vi "读D字符转数值.vi"(10 "读取D个数":i32=1 min=0 max=10, 11 "读取D地址":i32) -> (2 "读取的字节数":i32, 3 "连接的字符串":string)   [LabVIEW 2012]
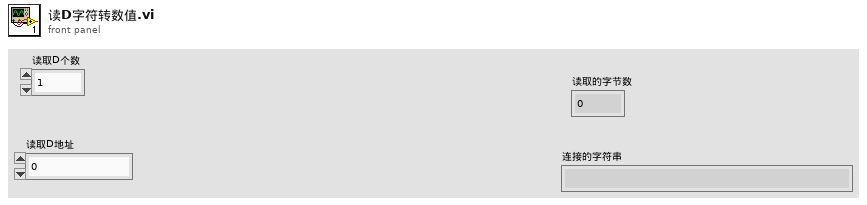
[diagram p1: front panel]
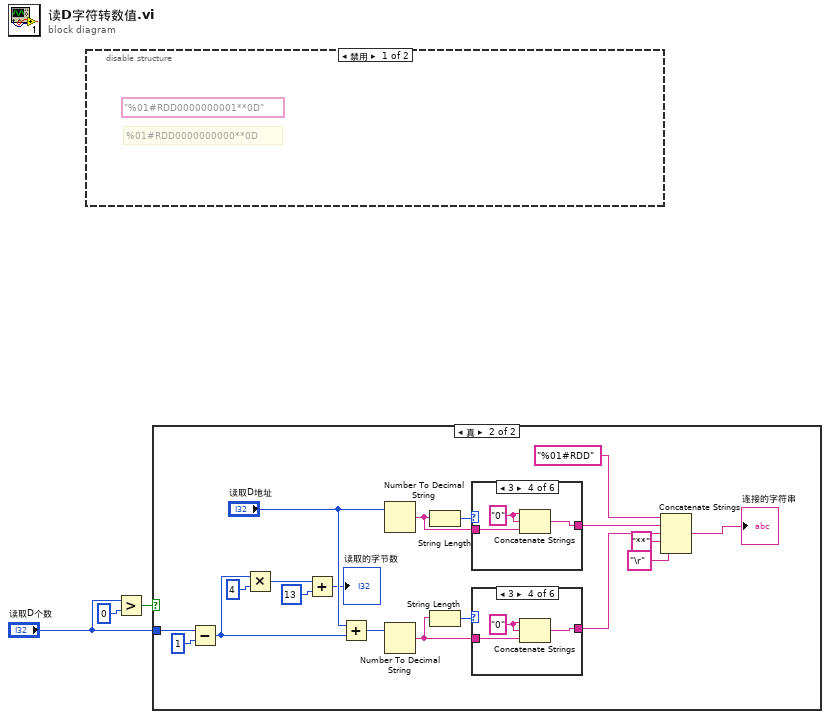
[diagram p0: block diagram]
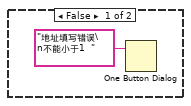
[diagram p2: hidden frame]
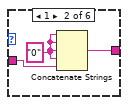
[diagram p4: hidden frame]
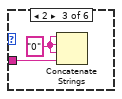
[diagram p5: hidden frame]
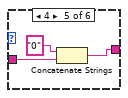
[diagram p6: hidden frame]
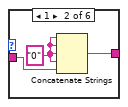
[diagram p9: hidden frame]
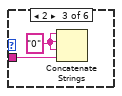
[diagram p10: hidden frame]
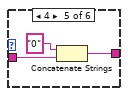
[diagram p11: hidden frame]
diagram:
  n1 = disable-structure shown="禁用" {
    frame Disabled {
      (unwired) "%01#RDD0000000001**0D" ("字符串")
      # "%01#RDD0000000000**0D"
    }
    frame Enabled {
    }
  }
  n2 = Greater?(x="读取D个数", y=0) -> (0:w2:bool)
  n3 = case shown="真" w2 {
    tunnel: "读取D个数" -> [_ w8]
    frame False {
      n4 = One Button Dialog(message="地址填写错误\n不能小于1  " ("消息")) -> ()  [unwired: 1 in, 1 out]
    }
    frame True {
      n5 = Subtract(x=w8, y=1) -> (x-y=w7:i32)
      n6 = Multiply(x=w7, y=4) -> (x*y=w15:i32)
      n7 = Add(x=w15, y=13) -> (x+y=→"读取的字节数":i32)
      n8 = Add(x="读取D地址", y=w7) -> (x+y=w18:i32)
      n9 = Number To Decimal String(number="读取D地址") -> (decimal integer string=w14:string)  [unwired: 1 in]
      n10 = Number To Decimal String(number=w18) -> (decimal integer string=w20:string)  [unwired: 1 in]
      n11 = String Length(string=w14) -> (length=w13:i32)
      n12 = String Length(string=w20) -> (length=w19:i32)
      n13 = case shown="3" w13 {
        tunnel: w14 -> [_ w38 w40 w43 w46 w47]
        tunnel: [_ w36 _ w41 w44 w47] -> w22
        frame 0, Default {
        }
        frame 1 {
          w37 = "0" ("字符串")
          n14 = Concatenate Strings(w37, w37, w37, w37, w38) -> (w36:string)
        }
        frame 2 {
          w39 = "0" ("字符串")
          n15 = Concatenate Strings(w39, w39, w39, w40) -> ()  [unwired: 1 out]
        }
        frame 3 {
          w42 = "0" ("字符串")
          n16 = Concatenate Strings(w42, w42, w43) -> (w41:string)
        }
        frame 4 {
          n17 = Concatenate Strings("0" ("字符串"), w46) -> (w44:string)
        }
        frame 5 {
        }
      }
      n18 = case shown="3" w19 {
        tunnel: w20 -> [_ w26 w28 w31 w34 w35]
        tunnel: [_ w24 _ w29 w32 w35] -> w23
        frame 0, Default {
        }
        frame 1 {
          w25 = "0" ("字符串")
          n19 = Concatenate Strings(w25, w25, w25, w25, w26) -> (w24:string)
        }
        frame 2 {
          w27 = "0" ("字符串")
          n20 = Concatenate Strings(w27, w27, w27, w28) -> ()  [unwired: 1 out]
        }
        frame 3 {
          w30 = "0" ("字符串")
          n21 = Concatenate Strings(w30, w30, w31) -> (w29:string)
        }
        frame 4 {
          n22 = Concatenate Strings("0" ("字符串"), w34) -> (w32:string)
        }
        frame 5 {
        }
      }
      n23 = Concatenate Strings("%01#RDD" ("字符串"), w22, w23, "**" ("字符串"), "\r" ("字符串")) -> (→"连接的字符串":string)
    }
  }
